vi "Export Instrument Addon Configuration.vi"(8 "error in (no error)":errorcluster, 10 "export file path":path, 11 "instrument addon refnum in":T1 format="%.0x") -> (0 "error out":errorcluster, 3 "instrument addon refnum out":T1 format="%.0x")   [LabVIEW 2019, in "Instrument Addon Scripting API.lvlib"]
doc: "Exports the configuration of a target Instrument Addon Custom Device to a .dat file. \nThis function will overwrite any existing .dat file at the target location."
uses:
  Instrument Addon Scripting API.lvlib
  <vilib>/NI VeriStand/Custom Device API/Custom Device Item Ref.ctl
  <vilib>/NI/NI VeriStand Custom Device Import and Export Tool/File Interface Class/File Interface.lvclass
  <vilib>/NI/NI VeriStand Custom Device Import and Export Tool/ImportExport.lvlib
  <vilib>/NI VeriStand/Custom Device API/Custom Device API.lvlib
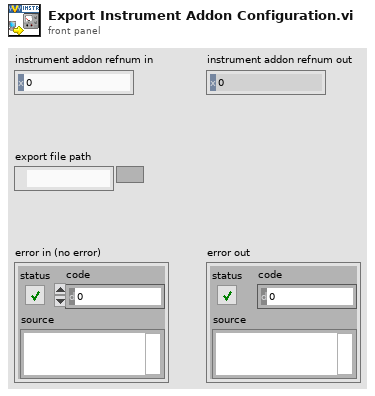
[diagram p1: front panel]
types:
  T1 = typedef "Custom Device API.lvlib/Custom Device Item Ref.ctl" = u64
  T2 = enum16{"open", "replace", "create", "open or create", "replace or create", "replace or create with confirmation"}
  T3 = typedef "Advanced System Definition.lvlib/SysDef.Export.ctl" = cluster{"Version":string, "Tree":T4[]}
  T4 = typedef "Advanced System Definition.lvlib/TreeItem.ctl" = cluster{"Item Info":T5, "Parent Path":string[], "Properties":T10[]}
  T5 = typedef "Advanced System Definition.lvlib/TreeItem.Info.ctl" = cluster{"Name":string, "Description":string, "GUID":string, "Is Channel":bool, "Channel":T6, "Is Waveform":bool, "Waveform":T8}
  T6 = typedef "Custom Device API.lvlib/Custom Device Channel.ctl" = cluster{"Type":T7, "Units":string, "Default Value":dbl, "Faultable":bool, "Scalable":bool}
  T7 = typedef "Custom Device API.lvlib/Custom Device Channel Type.ctl" = enum16{"Input", "Output"}
  T8 = typedef "Custom Device API.lvlib/Custom Device Waveform.ctl" = cluster{"Data Type":T9, "Units":string}
  T9 = typedef "Custom Device API.lvlib/Custom Device Waveform DataType.ctl" = enum16{"Double", "Complex Double"}
  T10 = typedef "Advanced System Definition.lvlib/TreeItem.Property.ctl" = cluster{"Name":string, "Type":i32, "Value":variant}
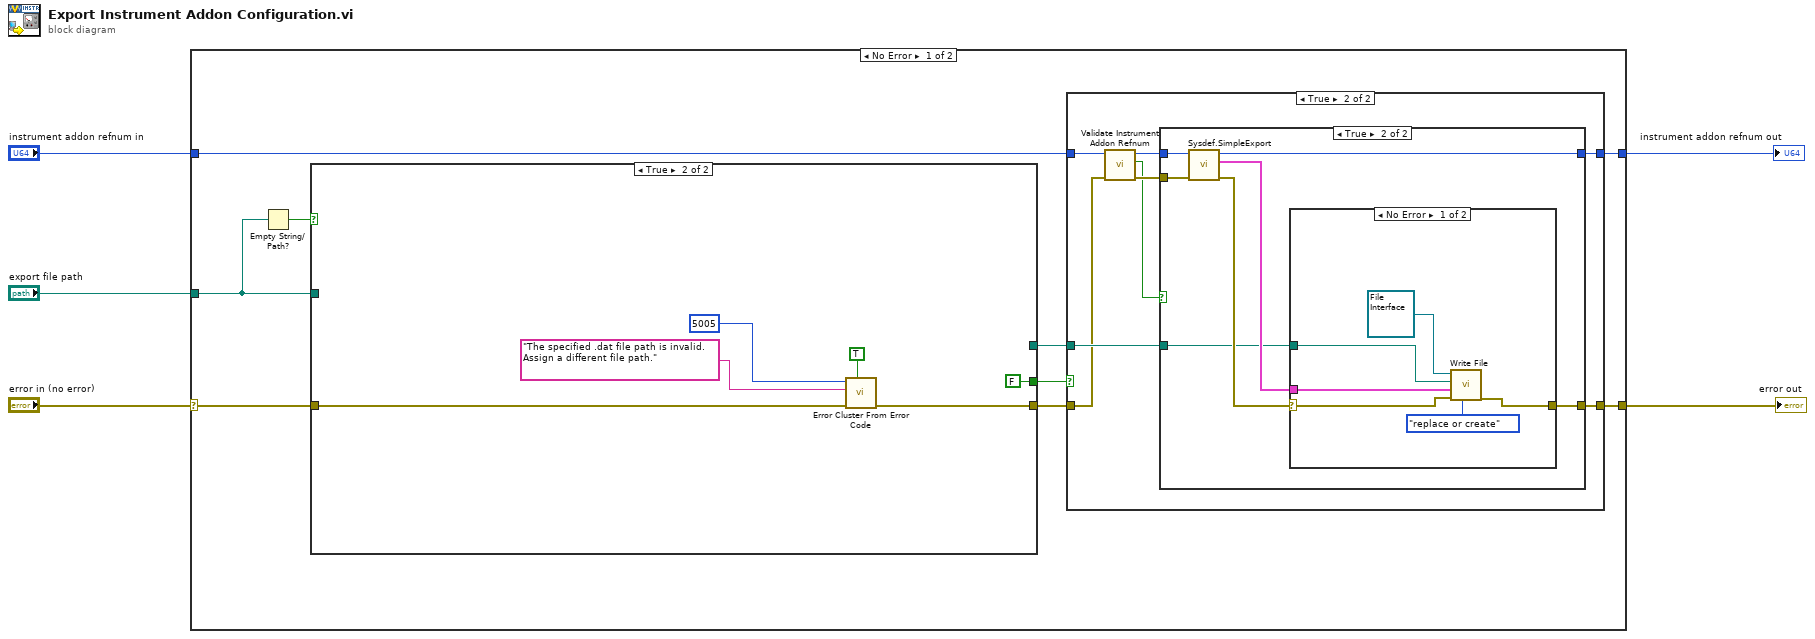
[diagram p0: block diagram]
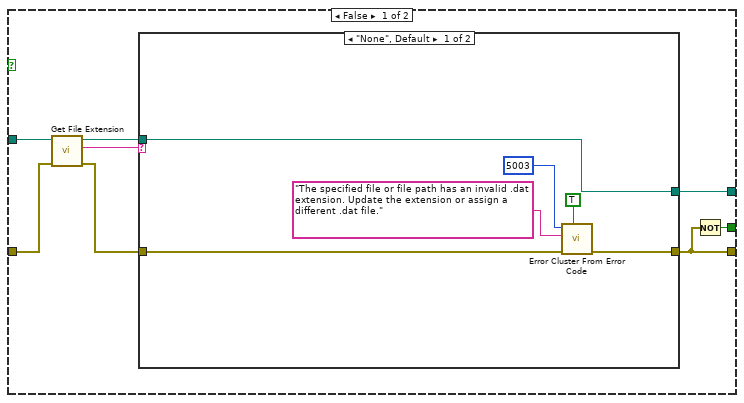
[diagram p5: hidden frame]
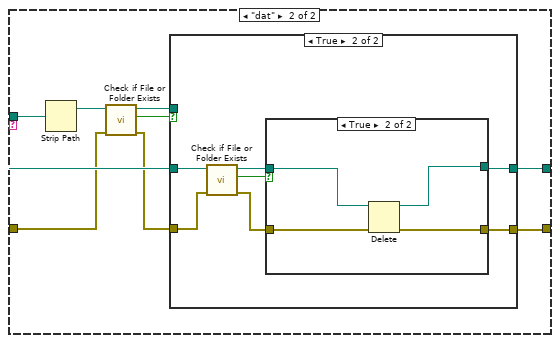
[diagram p6: hidden frame]
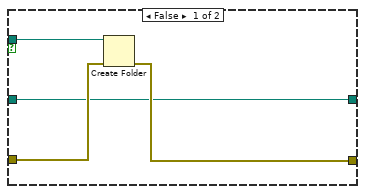
[diagram p7: hidden frame]
diagram:
  n1 = case shown="No Error" "error in (no error)" {
    selector: "error in (no error)" -> [w9 w86]
    tunnel: "instrument addon refnum in" -> [w14 w87]
    tunnel: [w13 w87] -> w1
    tunnel: [w12 w86] -> w5
    tunnel: "export file path" -> [w10 _]
    frame No Error {
      n2 = Empty String/Path?(string/path=w10) -> (empty?=w11:bool)
      n3 = case shown="True" w11 {
        tunnel: w9 -> [w48 w82]
        tunnel: w10 -> [w44 _]
        tunnel: [w42 w81] -> w7
        tunnel: [w43 _] -> w6
        tunnel: [w41 FALSE] -> w8
        frame False {
          n4 = call <vilib>:"Get File Extension.vi"("error in (no error)"=w48, "file"=w44) -> ("error out"=w47:errorcluster, "lowercase file extension"=w45:string, "dup file"=w46:path)  [unwired: 5 in, 2 out]
          n5 = case shown="\"None\", Default" w45 {
            tunnel: w47 -> [w52 w57]
            tunnel: w46 -> [w50 w59]
            tunnel: [w51 w55] -> w42
            tunnel: [w50 w58] -> w43
            frame "None", Default {
              n6 = call <vilib>:"Error Cluster From Error Code.vi"("show call chain? (False)"=TRUE, "error in (no error)"=w52, "error message (\"\")"="The specified file or file path has an invalid .dat extension. Update the extension or assign a different .dat file." ("error message (\"\")"), "error code (0)"=5003) -> ("error out"=w51:errorcluster)  [unwired: 5 in]
            }
            frame "dat" {
              n7 = Strip Path(path=w59) -> (stripped path=w62:path)  [unwired: 1 out]
              n8 = call <vilib>:"Check if File or Folder Exists.vi"("error in (no error)"=w57, "path"=w62) -> ("error out"=w56:errorcluster, "file or folder exists?"=w61:bool, "dup path"=w60:path)  [unwired: 7 in]
              n9 = case shown="True" w61 {
                tunnel: w56 -> [w66 w72]
                tunnel: w60 -> [w65 _]
                tunnel: [w64 w67] -> w55
                tunnel: w59 -> [w63 w70]
                tunnel: [w63 w68] -> w58
                frame False {
                  n10 = Create Folder(path (use dialog)=w65, error in=w66) -> (error out=w64:errorcluster)  [unwired: 1 in, 2 out]
                }
                frame True {
                  n11 = call <vilib>:"Check if File or Folder Exists.vi"("error in (no error)"=w72, "path"=w70) -> ("error out"=w71:errorcluster, "file or folder exists?"=w73:bool, "dup path"=w69:path)  [unwired: 7 in]
                  n12 = case shown="True" w73 {
                    tunnel: w71 -> [w75 w79]
                    tunnel: w69 -> [w74 w78]
                    tunnel: [w75 w77] -> w67
                    tunnel: [w74 w76] -> w68
                    frame False {
                    }
                    frame True {
                      n13 = Delete(path (use dialog)=w78, error in=w79) -> (deleted path=w76:path, error out=w77:errorcluster)  [unwired: 3 in, 1 out]
                    }
                  }
                }
              }
            }
          }
          n14 = Not(x=w42) -> (.not. x?=w41:bool)
        }
        frame True {
          n15 = call <vilib>:"Error Cluster From Error Code.vi"("show call chain? (False)"=TRUE, "error in (no error)"=w82, "error message (\"\")"="The specified .dat file path is invalid. Assign a different file path." ("error message (\"\")"), "error code (0)"=5005) -> ("error out"=w81:errorcluster)  [unwired: 5 in]
        }
      }
      n16 = case shown="True" w8 {
        tunnel: w14 -> [w16 w19]
        tunnel: [w16 w24] -> w13
        tunnel: [w15 w23] -> w12
        tunnel: w7 -> [w15 w21]
        tunnel: w6 -> [_ w22]
        frame False {
        }
        frame True {
          n17 = call "Validate Instrument Addon Refnum.vi"("Error In"=w21, "Refnum In"=w19) -> ("Error Out"=w20:errorcluster, "Is Instrument Addon?"=w17:bool, "Refnum Out"=w18:T1)  [unwired: 7 in]
          n18 = case shown="True" w17 {
            tunnel: [w26 w31] -> w24
            tunnel: [w25 w30] -> w23
            tunnel: w22 -> [_ w29]
            tunnel: w20 -> [w25 w28]
            tunnel: w18 -> [w26 w27]
            frame False {
            }
            frame True {
              n19 = call <vilib>:"Sysdef.SimpleExport.vi"("error in (no error)"=w28, "ID"=w27) -> ("error out"=w33:errorcluster, "Export"=w32:T3, "ID out"=w31:u64)  [unwired: 7 in]
              n20 = case shown="No Error" w33 {
                selector: w33 -> [w37 w40]
                tunnel: [w38 w40] -> w30
                tunnel: w32 -> [w39 _]
                tunnel: w29 -> [w36 _]
                frame No Error {
                  n21 = call-dynamic "Write File.vi"("operation"=T2."replace or create", "error in (no error)"=w37, "Data"=w39, "datalog path (use dialog)"=w36, "File Interface in"=refnum<class "File Interface.lvclass"> refnum) -> ("error out"=w38:errorcluster)  [unwired: 6 in]
                }
                frame Error {
                }
              }
            }
          }
        }
      }
    }
    frame Error {
    }
  }
  "error out" <- w5
  "instrument addon refnum out" <- w1
